vi "ConnectionManager.vi"(0 "STOMP In":refnum<class "STOMP.lvclass">, 1 "address":string="localhost", 2 "port":u16=61613, 5 "error in (no error)":errorcluster) -> (19 "error out":errorcluster)   [LabVIEW 2017, in "STOMP.lvclass"]
uses:
  STOMP.lvclass
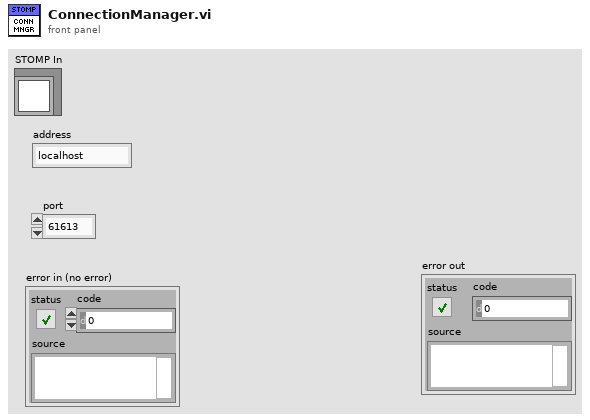
[diagram p1: front panel]
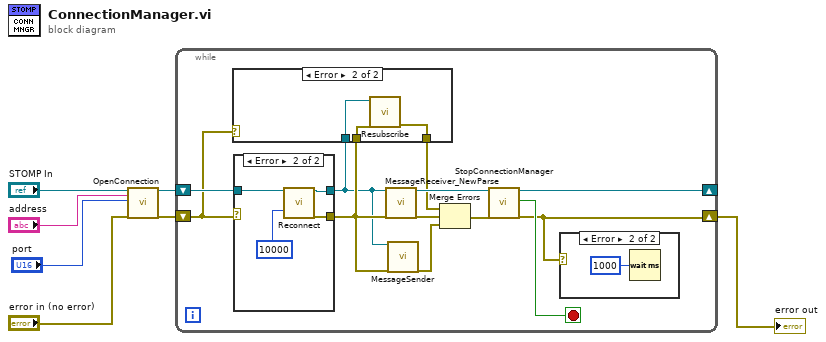
[diagram p0: block diagram]
diagram:
  n1 = call-dynamic "OpenConnection.vi"("STOMP in"="STOMP In", "address"="address", "port"="port", "error in (no error)"="error in (no error)") -> ("STOMP out"=w6:refnum<class "STOMP.lvclass">, "error out"=w5:errorcluster)  [unwired: 14 in]
  n2 = while {
    shift-right: [w12] -> w7
    shift-left: w5 -> [w10]
    shift-right: [w13] -> _
    shift-left: w6 -> [w19]
    stop <- w16 stop-if-true
    n3 = case shown="Error" w10 {
      selector: w10 -> [w25 _]
      tunnel: [w26 w29] -> w8
      tunnel: w19 -> [w26 w30]
      tunnel: [w25 w28] -> w9
      frame No Error {
      }
      frame Error {
        n4 = call-dynamic "Reconnect.vi"("STOMP in"=w30, "timeout ms (10000)"=10000 ("timeout ms (60000)")) -> ("STOMP out"=w29:refnum<class "STOMP.lvclass">, "error out"=w28:errorcluster)  [unwired: 16 in]
      }
    }
    n5 = case shown="Error" w10 {
      tunnel: [w20 w23] -> w11
      tunnel: w9 -> [w20 w22]
      tunnel: w8 -> [_ w21]
      frame No Error {
      }
      frame Error {
        n6 = call-dynamic "Resubscribe.vi"("error in (no error)"=w22, "STOMP in"=w21) -> ("error out"=w23:errorcluster)  [unwired: 8 in, 1 out]
      }
    }
    n7 = call "MessageReceiver_NewParse.vi"("STOMP In"=w8, "error in (no error)"=w9) -> ("STOMP out"=w17:refnum<class "STOMP.lvclass">, "error out"=w18:errorcluster)  [unwired: 16 in]
    n8 = call "MessageSender.vi"("STOMP In"=w8, "error in (no error)"=w9) -> ("error out"=w14:errorcluster)  [unwired: 16 in, 1 out]
    n9 = Merge Errors(w11, w18, w14) -> (w15:errorcluster)
    n10 = call-dynamic "StopConnectionManager.vi"("STOMP in"=w17, "error in (no error)"=w15) -> ("STOMP out"=w13:refnum<class "STOMP.lvclass">, "stop?"=w16:bool, "error out"=w12:errorcluster)  [unwired: 15 in]
    n11 = case shown="Error" w12 {
      frame No Error {
      }
      frame Error {
        n12 = Wait (ms)(milliseconds to wait=u32 1000) -> ()  [unwired: 1 out]
      }
    }
  }
  "error out" <- w7
